vi "Write Config.vi"(8 "error in (no error)":errorcluster, 9 "Re-Init?":bool, 10 "ICM File In":path, 11 "Query in":refnum<class "Query.lvclass">) -> (0 "error out":errorcluster, 3 "Query out":refnum<class "Query.lvclass">)   [LabVIEW 2024, in "Query.lvclass"]
doc: "Query.lvclass:Write Config.vi\n\nThis is the template for the Write Config VI for the Query class.\n\nInstrument Communication Module Version 1.0\nSeptember, 2017 Original Code Consulting David Thomson\n www.originalcode.com"
uses:
  Query.lvclass
  Query.lvclass/Query.ctl
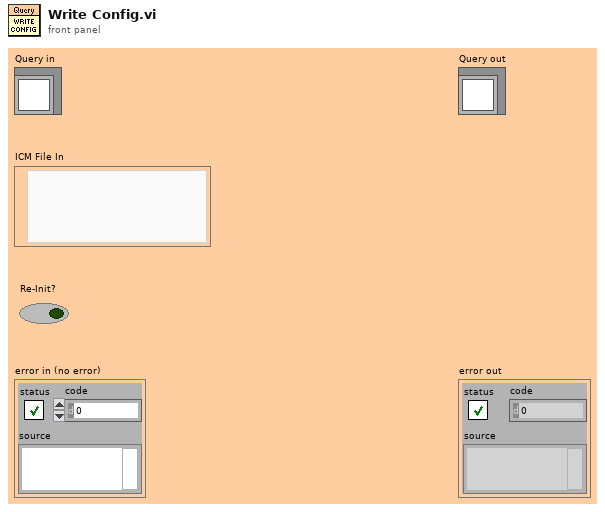
[diagram p1: front panel]
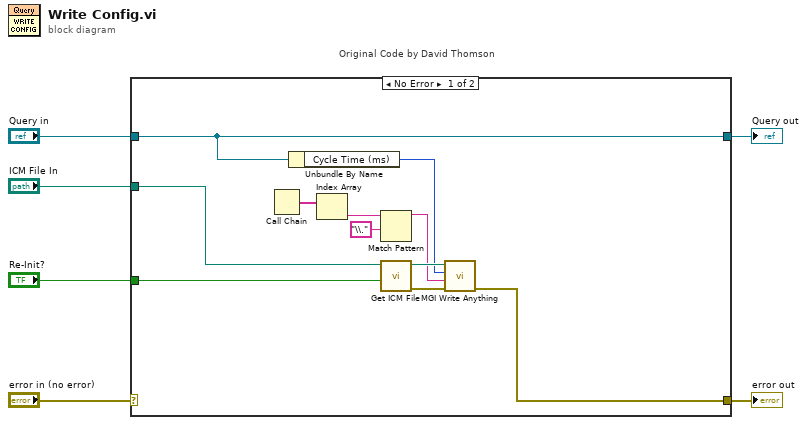
[diagram p0: block diagram]
diagram:
  n1 = case "Original Code by David Thomson" shown="No Error" "error in (no error)" {
    selector: "error in (no error)" -> [_ w19]
    tunnel: [w10 w19] -> w5
    tunnel: [w7 w18] -> w3
    tunnel: "Query in" -> [w7 w18]
    tunnel: "Re-Init?" -> [w9 _]
    tunnel: "ICM File In" -> [w8 _]
    frame No Error {
      n2 = Call Chain() -> (call chain=w16:string[])
      n3 = Unbundle By Name(w7) -> ("Cycle Time (ms)"=w11:u32)
      n4 = Index Array(array=w16) -> (element=w15:string)  [unwired: 1 in]
      n5 = Match Pattern(string=w15, regular expression="\\.") -> (before substring=w12:string)  [unwired: 1 in, 3 out]
      n6 = call "Get ICM File.vi"("Re-Init?"=w9, "ICM File In"=w8) -> ("error out"=w14:errorcluster, "ICM File"=w13:path)  [unwired: 8 in]
      n7 = call "MGI Write Anything.vi"("Error In"=w14, "Section Name (Name of \"Anything\")"=w12, "Anything"=w11, "Path (dialog)"=w13) -> ("Error Out"=w10:errorcluster)  [unwired: 5 in, 2 out]
    }
    frame Error {
    }
  }
  "error out" <- w5
  "Query out" <- w3
